vi "SVT Initialize Waterfall Display for Octave.vi"(0 "window title":string="Waterfall", 5 "display bounds":T1={"left"=20, "top"=20, "width"=600, "height"=400} {"height" min=300; "width" min=400}, 7 "number of plots":i32, 11 "error in (no error)":errorcluster, 12 "colors":T2={"frame"=16763904, "plot"=52224, "background"=0}) -> (4 "waterfall ref":refnum<vi>, 15 "error out":errorcluster)   [LabVIEW 2017]
doc: "Initializes the waterfall display for octave spectra and generates the waterfall reference used to send data to the display or to close the display."
uses:
  <vilib>/addons/Sound and Vibration/compatibility/Waterfall/subVIs/sv_Waterfall for Octave Global.vi
panel:
  in  "invalid waterfall ref":refnum<vi>
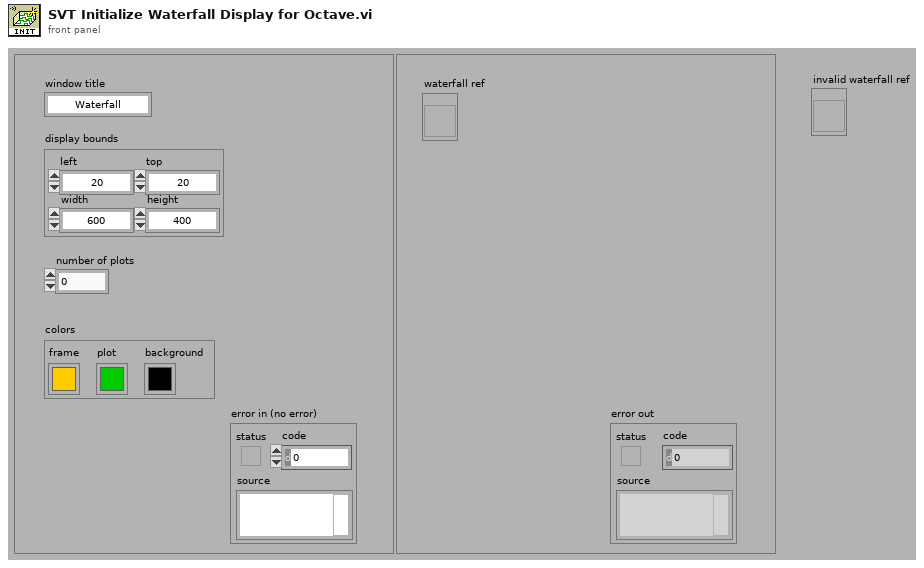
[diagram p1: front panel]
types:
  T1 = cluster{"left":i16, "top":i16, "width":i16, "height":i16}
  T2 = cluster{"frame":u32, "plot":u32, "background":u32}
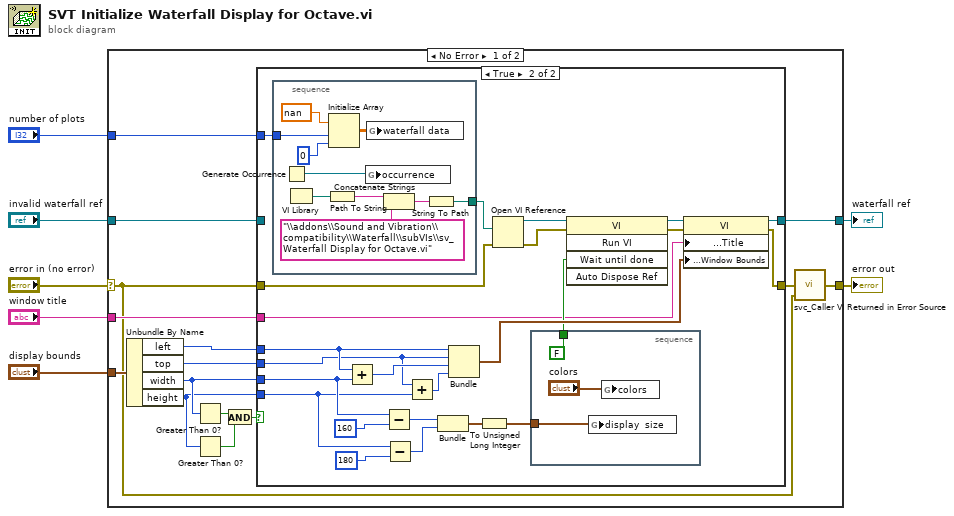
[diagram p0: block diagram]
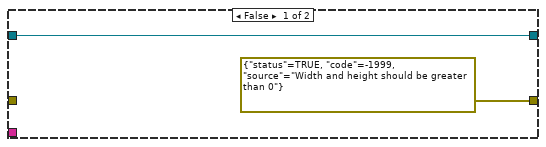
[diagram p2: hidden frame]
diagram:
  n1 = case shown="No Error" "error in (no error)" {
    selector: "error in (no error)" -> [w8 w63]
    tunnel: [w22 w62] -> w7
    tunnel: [w18 w63] -> w6
    tunnel: "window title" -> [w17 _]
    tunnel: "display bounds" -> [w16 _]
    tunnel: "invalid waterfall ref" -> [w15 w62]
    tunnel: "number of plots" -> [w9 _]
    frame No Error {
      n2 = Unbundle By Name(w16) -> ("left"=w21:i16, "top"=w20:i16, "width"=w14:i16, "height"=w13:i16)
      n3 = Greater Than 0?(x=w14) -> (x > 0?=w12:bool)
      n4 = Greater Than 0?(x=w13) -> (x > 0?=w11:bool)
      n5 = And(x=w12, y=w11) -> (x .and. y?=w10:bool)
      n6 = case shown="True" w10 {
        tunnel: [w24 w45] -> w22
        tunnel: w21 -> [_ w43]
        tunnel: w20 -> [_ w41]
        tunnel: w14 -> [_ w37]
        tunnel: w13 -> [_ w33]
        tunnel: [errorcluster {"status"=TRUE, "code"=-1999, "source"="Width and height should be greater than 0"} ("Error IO") w31] -> w19
        tunnel: w8 -> [_ w27]
        tunnel: w17 -> [_ w26]
        tunnel: w15 -> [w24 _]
        tunnel: w9 -> [_ w25]
        frame False {
        }
        frame True {
          n7 = stacked-sequence {
            tunnel: [w53] -> w29
            tunnel: w25 -> [w50]
            frame #0 {
              n8 = Generate Occurrence() -> (w58:refnum<k4>)
              n9 = VI Library() -> (path=w54:path)
              n10 = Path To String(path=w54) -> (string=w57:string)
              n11 = Initialize Array(nan ("element"), w50, 0 ("dimension size")) -> (w49:dbl[][])
              n12 = global write "sv_Waterfall for Octave Global.vi" "occurrence"(w58) -> ()
              n13 = global write "sv_Waterfall for Octave Global.vi" "waterfall data"(w49) -> ()
              n14 = Concatenate Strings(w57, "\\addons\\Sound and Vibration\\compatibility\\Waterfall\\subVIs\\sv_Waterfall Display for Octave.vi" ("Substring")) -> (w55:string)
              n15 = String To Path(string=w55) -> (path=w53:path)
            }
          }
          n16 = Add(x=w43, y=w37) -> (x+y=w42:i16)
          n17 = Subtract(x=w37, y=i16 160) -> (x-y=w35:i16)
          n18 = Subtract(x=w33, y=i16 180) -> (x-y=w32:i16)
          n19 = Add(x=w41, y=w33) -> (x+y=w40:i16)
          n20 = Bundle(w35, w32) -> (w39:cluster{i16, i16})  [unwired: 1 in]
          n21 = Bundle("left"=w43, "top"=w41, w42, w40) -> (w44:cluster{"left":i16, "top":i16, i16, i16})  [unwired: 1 in]
          n22 = To Unsigned Long Integer(number=w39) -> (unsigned 32bit integer=w38:cluster{u32, u32})
          n23 = Open VI Reference(vi path=w29, error in (no error)=w27) -> (vi reference=w28:refnum<vi>, error out=w48:errorcluster)  [unwired: 4 in]
          n24 = stacked-sequence {
            tunnel: w38 -> [w60]
            tunnel: [FALSE ("Wait until done")] -> w30
            frame #0 {
              n25 = global write "sv_Waterfall for Octave Global.vi" "display  size"(w60) -> ()
              n26 = global write "sv_Waterfall for Octave Global.vi" "colors"("colors") -> ()
            }
          }
          n27 = invoke class="VI" method="Run VI"(reference=w28, error in=w48, "Wait until done"=w30) -> (reference out=w46:refnum<vi>, error out=w47:errorcluster)  [unwired: 2 in, 3 out]
          n28 = property class="VI"(reference=w46, error in=w47, "Front Panel Window:Title"=w26, "Front Panel Window:Window Bounds"=w44) -> (reference out=w45:refnum<vi>, error out=w31:errorcluster)
        }
      }
      n29 = call <vilib>:"svc_Caller VI Returned in Error Source.vi"("warning input to caller"=w8, "error in (no error)"=w19) -> ("error out"=w18:errorcluster)  [unwired: 3 in]
    }
    frame Error {
    }
  }
  "error out" <- w6
  "waterfall ref" <- w7
